vi "Check Escala.vi"(8 "error in (no error)":errorcluster, 10 "Grandeza":string, 11 "U1252 in":refnum<class "U1252.lvclass">) -> (0 "error out":errorcluster, 2 "Escala Correta?":bool, 3 "U1252 out":refnum<class "U1252.lvclass">)   [LabVIEW 2015, in "U1252.lvclass"]
uses:
  U1252.lvclass
  <instrlib>/U1250 Series Multimeter Device Driver/U1250 Series Digital Multimeter.lvlib
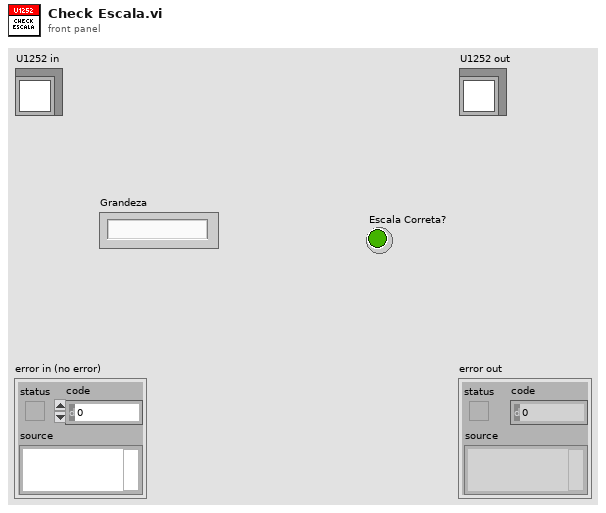
[diagram p1: front panel]
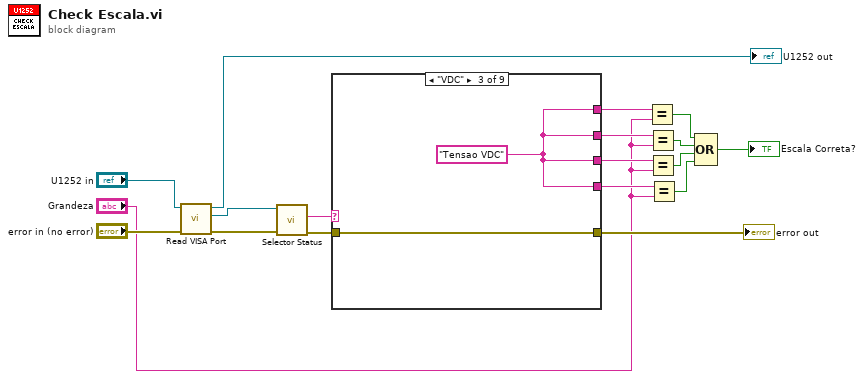
[diagram p0: block diagram]
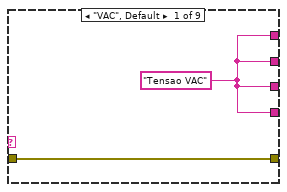
[diagram p2: hidden frame]
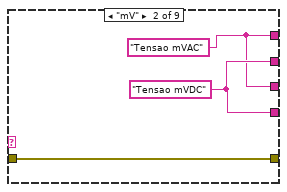
[diagram p3: hidden frame]
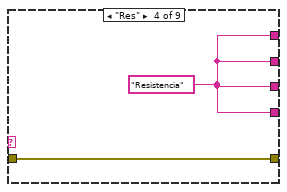
[diagram p4: hidden frame]
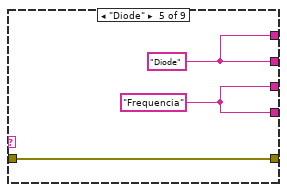
[diagram p5: hidden frame]
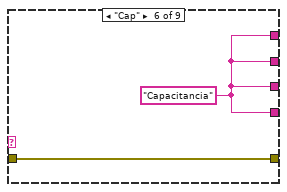
[diagram p6: hidden frame]
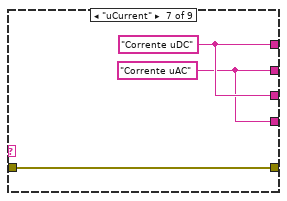
[diagram p7: hidden frame]
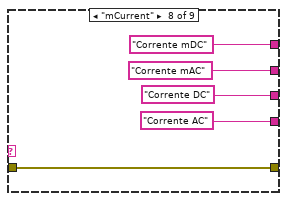
[diagram p8: hidden frame]
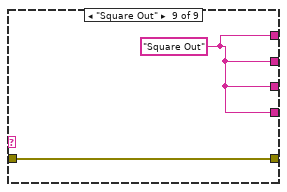
[diagram p9: hidden frame]
diagram:
  n1 = call-dynamic "Read VISA Port.vi"("error in (no error)"="error in (no error)", "Device in"="U1252 in") -> ("error out"=w16:errorcluster, "VISA Port"=w1:refnum<visa-resource-name>, "Device out"=→"U1252 out":refnum<class "U1252.lvclass">)  [unwired: 7 in]
  n2 = call <instrlib>:"Selector Status.vi"("error in (no error)"=w16, "VISA resource name"=w1) -> ("error out"=w11:errorcluster, "Selector Option"=w14:string)  [unwired: 7 in, 1 out]
  n3 = case shown="\"VDC\"" w14 {
    tunnel: [w19 w22 w24 w26 w29 w31 w33 "Corrente mAC" w41] -> w13
    tunnel: [w20 w23 w25 w27 w30 w32 w35 w39 w42] -> w12
    tunnel: w11 -> [w20 w23 w25 w27 w30 w32 w35 w39 w42]
    tunnel: [w19 w21 w24 w26 w29 w31 w34 "Corrente mDC" w41] -> w8
    tunnel: [w19 w21 w24 w26 w28 w31 w34 "Corrente DC" w41] -> w6
    tunnel: [w19 w22 w24 w26 w28 w31 w33 "Corrente AC" w41] -> w5
    frame "VAC", Default {
      w19 = "Tensao VAC"
    }
    frame "mV" {
      w21 = "Tensao mVAC"
      w22 = "Tensao mVDC"
    }
    frame "VDC" {
      w24 = "Tensao VDC"
    }
    frame "Res" {
      w26 = "Resistencia"
    }
    frame "Diode" {
      w28 = "Frequencia"
      w29 = "Diode"
    }
    frame "Cap" {
      w31 = "Capacitancia"
    }
    frame "uCurrent" {
      w34 = "Corrente uDC"
      w33 = "Corrente uAC"
    }
    frame "mCurrent" {
    }
    frame "Square Out" {
      w41 = "Square Out"
    }
  }
  "error out" <- w12
  n4 = Equal?(x=w8, y="Grandeza") -> (x = y?=w9:bool)
  n5 = Equal?(x=w13, y="Grandeza") -> (x = y?=w7:bool)
  n6 = Equal?(x=w6, y="Grandeza") -> (x = y?=w2:bool)
  n7 = Equal?(x=w5, y="Grandeza") -> (x = y?=w3:bool)
  n8 = Compound Arithmetic op=OR(w9, w7, w2, w3) -> (→"Escala Correta?":bool)
